vi "PH_Waveplate-GUI_6P.Set Position to GUI.vi"(0 "i ref in":refnum<vi>, 2 "Axis Information":T1, 3 "no link":bool, 5 "error in":errorcluster) -> (14 "i ref out":refnum<vi>, 19 "error out":errorcluster)   [LabVIEW 2014, in "PH_Waveplate-GUI_6P.lvlib"]
uses:
  PH_Waveplate-GUI_6P.lvlib
  PH_Stepmotor_BaseClass/PH_Stepmotor_BaseClass.Axis Information.ctl
  PH_Stepmotor_BaseClass/PH_Stepmotor_BaseClass.Axis Activity.ctl
  PH_Stepmotor_BaseClass/PH_Stepmotor_BaseClass.lvlib
  PH_Common/PH_Common.lvlib
  PH_AxisGUI_BaseClass/PH_AxisGUI_BaseClass.lvlib
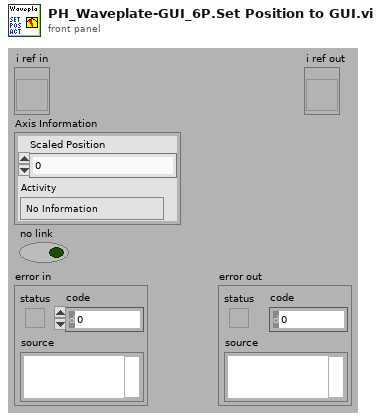
[diagram p1: front panel]
types:
  T1 = typedef "PH_Stepmotor_BaseClass.lvlib/PH_Stepmotor_BaseClass.Axis Information.ctl" = cluster{"Scaled Position":dbl, "Activity":T2}
  T2 = typedef "PH_Stepmotor_BaseClass.lvlib/PH_Stepmotor_BaseClass.Axis Activity.ctl" = enum16{"No Information", "stopped", "running", "Failure", "Alarm", "stopped at backward ES", "stopped at foreward ES"}
  T3 = enum8{"Enabled", "Disabled", "Disabled and Grayed Out"}
  T4 = typedef "PH_AxisGUI_BaseClass.lvlib/PH_AxisGUI_BaseClass.i attribute.ctl" = cluster{"Axes":T5[]}
  T5 = typedef "PH_AxisGUI_BaseClass.lvlib/PH_AxisGUI_BaseClass.Axis Attributes.ctl" = cluster{"Axis GUI Refs":T6, "Address":T7, "Name":string, "Label \"Back\"":string, "Labell \"Forth\"":string, "Moving?":bool}
  T6 = typedef "PH_AxisGUI_BaseClass.lvlib/PH_AxisGUI_BaseClass.Axis GUI Refs.ctl" = cluster{"Back":refnum<vi>, "Forth":refnum<vi>, "Status":refnum<vi>, "Target":refnum<vi>, "Address":refnum<vi>, "Status Bar":refnum<vi>, "Settings":refnum<vi>, "Activity":refnum<vi>, "Clear Error":refnum<vi>}
  T7 = typedef "PH_Stepmotor_BaseClass.lvlib/PH_Stepmotor_BaseClass.Axis Address.ctl" = cluster{"Instance":string, "Motor Nr":i32}
  T8 = typedef "PH_Waveplate-GUI_6P.lvlib/PH_Waveplate-GUI_6P.i attribute.ctl" = cluster{"GUI Refs":cluster{"Meter":refnum<vi>, "Extend Limits":refnum<vi>, "Type":refnum<vi>, "Target":refnum<vi>}, "Extend Waveplate Limit":bool, "Type":T9, "Limit":dbl}
  T9 = typedef "PH_Waveplate-GUI_6P.lvlib/PH_Waveplate-GUI_6P.Type.ctl" = u16
  T10 = typedef "PH_Stepmotor_BaseClass.lvlib/PH_Stepmotor_BaseClass.Axis Settings.ctl" = cluster{"Sign change":bool, "Width":dbl, "Calibration":dbl, "Unit":string, "Motor Type":T11, "Unit Width":string, "Unit CF":string}
  T11 = typedef "PH_Stepmotor_BaseClass.lvlib/PH_Stepmotor_BaseClass.Motor Type.ctl" = enum16{"Unspecific", "OWIS 49.120.2633", "OWIS 49.060.1033", "OWIS 43.040.2558", "Diamond Motion 2200 series", "OWIS 49.120.266B.MV6", "Calorimeter", "Linear Stage 1", "MICOS VT-80", "MICOS VT-80 S", "Standa Rotstage nt0.95A", "PUF RA 320.200", "PUF RA 800.200", "PUF RA 800.400", "PUF RA 400.50", "1324.nn.800.50", "1324.n9c.800.50", "1324.nn.320.200", "1324.nn.400.200", "1324.nn.800.200", "1324.nn.400.50", "1324.8c9c.800.50", "1324.8c9c.400.200"}
  T12 = cluster{"rel. Intensity [%]":dbl, "rel. Intensity [%]":dbl}
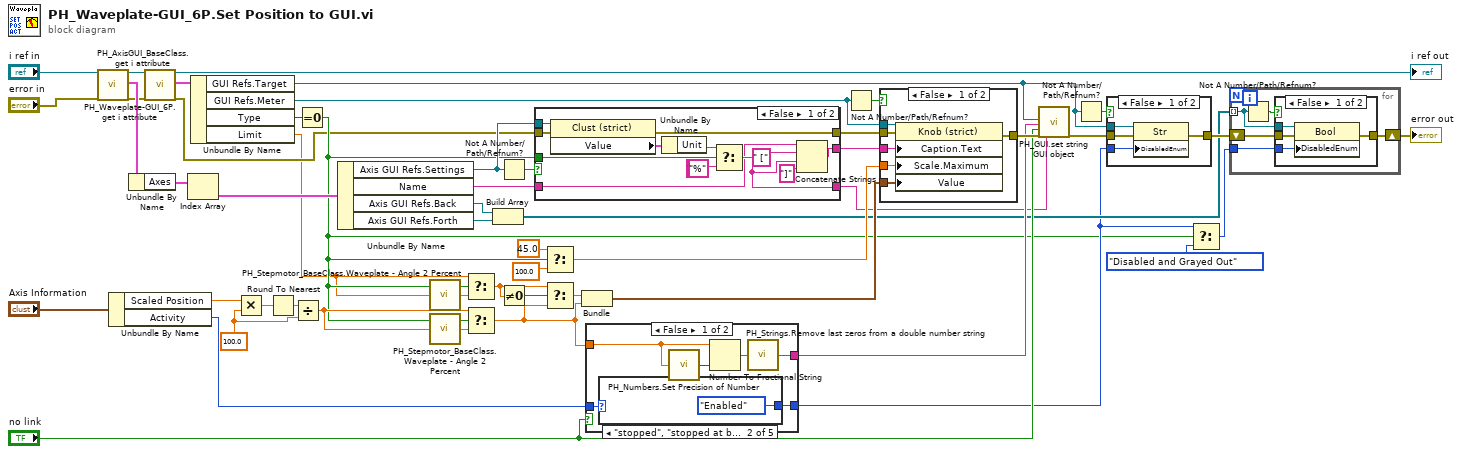
[diagram p0: block diagram]
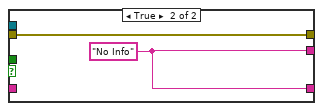
[diagram p3: hidden frame]
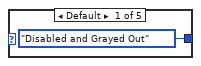
[diagram p5: hidden frame]
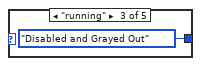
[diagram p6: hidden frame]
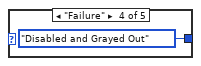
[diagram p7: hidden frame]
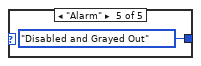
[diagram p8: hidden frame]
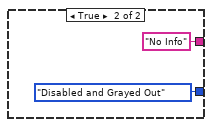
[diagram p9: hidden frame]
diagram:
  w46 = 100.0 ("x")
  n1 = call "PH_AxisGUI_BaseClass.get i attribute.vi"("i ref in"="i ref in", "error in (no error)"="error in") -> ("i ref out"=w14:refnum<vi>, "i attribute"=w27:T4, "error out"=w13:errorcluster)  [unwired: 15 in]
  n2 = Unbundle By Name("Axis Information") -> ("Scaled Position"=w31:dbl, "Activity"=w30:T2)
  n3 = Unbundle By Name(w27) -> ("Axes"=w26:T5[])
  n4 = call "PH_Waveplate-GUI_6P.get i attribute.vi"("i ref in"=w14, "error in (no error)"=w13) -> ("i ref out"=→"i ref out":refnum<vi>, "i attribute"=w51:T8, "error out"=w4:errorcluster)  [unwired: 15 in]
  n5 = Index Array(array=w26) -> (element=w25:T5)  [unwired: 1 in]
  n6 = Unbundle By Name(w51) -> ("GUI Refs.Target"=w34:refnum<vi>, "GUI Refs.Meter"=w50:refnum<vi>, "Type"=w44:T9, "Limit"=w3:dbl)
  n7 = Multiply(x=w31, y=w46) -> (x*y=w48:dbl)
  n8 = Round To Nearest(number=w48) -> (nearest integer value=w47:dbl)
  n9 = Divide(x=w47, y=w46) -> (x/y=w43:dbl)
  n10 = Equal To 0?(x=w44) -> (x = 0?=w6:bool)
  n11 = Unbundle By Name(w25) -> ("Axis GUI Refs.Settings"=w16:refnum<vi>, "Name"=w15:string, "Axis GUI Refs.Back"=w11:refnum<vi>, "Axis GUI Refs.Forth"=w12:refnum<vi>)
  n12 = call "PH_Stepmotor_BaseClass.Waveplate - Angle 2 Percent.vi"("Angle [°]"=w3) -> ("rel. Intensity [%]"=w40:dbl)
  n13 = call "PH_Stepmotor_BaseClass.Waveplate - Angle 2 Percent.vi"("Angle [°]"=w43) -> ("rel. Intensity [%]"=w42:dbl)
  n14 = Select(t=w3, s=w6, f=w40) -> (s? t:f=w41:dbl)
  n15 = Select(t=w43, s=w6, f=w42) -> (s? t:f=w23:dbl)
  n16 = Build Array(w11, w12) -> (w9:refnum<vi>[])
  n17 = Not A Number/Path/Refnum?(number/path/refnum=w16) -> (NaN/Path/Refnum?=w28:bool)
  n18 = Not Equal To 0?(x=w41) -> (x != 0?=w45:bool)
  n19 = case shown="False" w28 {
    tunnel: w16 -> [w61 _]
    tunnel: w4 -> [w54 w66]
    tunnel: [w56 w66] -> w20
    tunnel: w15 -> [w53 _]
    tunnel: [w58 w65] -> w10
    tunnel: [w57 w65] -> w24
    tunnel: w6 -> [w55 _]
    frame False {
      (unwired) "%" ("Unit")
      n20 = property class="Clust (strict)"(reference=w61, error in=w54) -> (error out=w56:errorcluster, "Value"=w60:T10)  [unwired: 1 out]
      n21 = Unbundle By Name(w60) -> ("Unit"=w59:string)
      n22 = Select(t=w59, s=w55, f="%" ("Unit")) -> (s? t:f=w58:string)
      n23 = Concatenate Strings(w53, " [" ("string"), w58, "]" ("string")) -> (w57:string)
    }
    frame True {
      w65 = "No Info"
    }
  }
  n24 = Select(t=45.0, s=w6, f=100.0) -> (s? t:f=w37:dbl)
  n25 = Select(t=w41, s=w45, f=w23) -> (s? t:f=w22:dbl)
  n26 = Bundle("rel. Intensity [%]"=w22, "rel. Intensity [%]"=w23) -> (w21:T12)  [unwired: 1 in]
  n27 = case shown="False" "no link" {
    tunnel: w30 -> [w72 _]
    tunnel: [w71 T3."Disabled and Grayed Out" ("f")] -> w7
    tunnel: [w69 "No Info"] -> w29
    tunnel: w23 -> [w68 _]
    frame False {
      n28 = case shown="\"stopped\", \"stopped at backward ES\", \"stopped at foreward ES\"" w72 {
        tunnel: [T3."Disabled and Grayed Out" ("f") T3."Enabled" ("f") T3."Disabled and Grayed Out" ("f") T3."Disabled and Grayed Out" ("f") T3."Disabled and Grayed Out" ("f")] -> w71
        frame Default {
        }
        frame "stopped", "stopped at backward ES", "stopped at foreward ES" {
        }
        frame "running" {
        }
        frame "Failure" {
        }
        frame "Alarm" {
        }
      }
      n29 = call "PH_Numbers.Set Precision of Number.vi"("Number"=w68) -> ("Precision"=w67:i16)
      n30 = Number To Fractional String(number=w68, precision (6)=w67) -> (F-format string=w70:string)  [unwired: 2 in]
      n31 = call "PH_Strings.Remove last zeros from a double number string.vi"("String in"=w70) -> ("String out"=w69:string)
    }
    frame True {
    }
  }
  n32 = Not A Number/Path/Refnum?(number/path/refnum=w50) -> (NaN/Path/Refnum?=w52:bool)
  n33 = case shown="False" w52 {
    tunnel: w20 -> [w83 w86]
    tunnel: w50 -> [w84 _]
    tunnel: [w85 w86] -> w36
    tunnel: w37 -> [w82 _]
    tunnel: w24 -> [w81 _]
    tunnel: w21 -> [w80 _]
    frame False {
      n34 = property class="Knob (strict)"(reference=w84, error in=w83, "Caption.Text"=w81, "Scale.Maximum"=w82, "Value"=w80) -> (error out=w85:errorcluster)  [unwired: 1 out]
    }
    frame True {
    }
  }
  n35 = call "PH_GUI.set string GUI object.vi"("GUI object Ref"=w34, "Text"=w29, "Blinking? (false)"="no link", "error in"=w36, "Caption (N/A)"=w10) -> ("error out"=w35:errorcluster)  [unwired: 14 in]
  n36 = Not A Number/Path/Refnum?(number/path/refnum=w34) -> (NaN/Path/Refnum?=w33:bool)
  n37 = case shown="False" w33 {
    tunnel: w35 -> [w90 w91]
    tunnel: [w89 w91] -> w19
    tunnel: w34 -> [w88 _]
    tunnel: w7 -> [w87 _]
    frame False {
      n38 = property class="Str"(reference=w88, error in=w90, "DisabledEnum"=w87) -> (error out=w89:errorcluster)  [unwired: 1 out]
    }
    frame True {
    }
  }
  n39 = Select(t=w7, s=w6, f=T3."Disabled and Grayed Out" ("Disabled")) -> (s? t:f=w5:T3)
  n40 = for {
    tunnel: w9 -> [w93] mode=indexing
    shift-right: [w95] -> w18
    shift-left: w19 -> [w96]
    tunnel: w5 -> [w92]
    n41 = Not A Number/Path/Refnum?(number/path/refnum=w93) -> (NaN/Path/Refnum?=w94:bool)
    n42 = case shown="False" w94 {
      tunnel: w96 -> [w99 w101]
      tunnel: [w100 w101] -> w95
      tunnel: w93 -> [w98 _]
      tunnel: w92 -> [w97 _]
      frame False {
        n43 = property class="Bool"(reference=w98, error in=w99, "DisabledEnum"=w97) -> (error out=w100:errorcluster)  [unwired: 1 out]
      }
      frame True {
      }
    }
  }
  "error out" <- w18
